vi "loopback.vi"() -> ()   [LabVIEW 2019]
uses:
  <vilib>/nican/nican.llb/ncNetAttr.ctl
panel:
  out "Output Array":string[][](table)
  in  "interface":string(combo)="CAN1"
  in  "stop":bool
  in  "Data":u8[](array[numeric])=[1, 2, 3, 4, 5, 6, 7, 8] format="%.0x"
  in  "Set RTR flag?":bool
  in  "Data Length":u32=8 max=8 format="%.0x"
  in  "Arbitration Id":u32=8 format="%.0x"
  in  "Write frame":bool
  in  "Baudrate":u32=125000
  # "Writing on CAN bus"
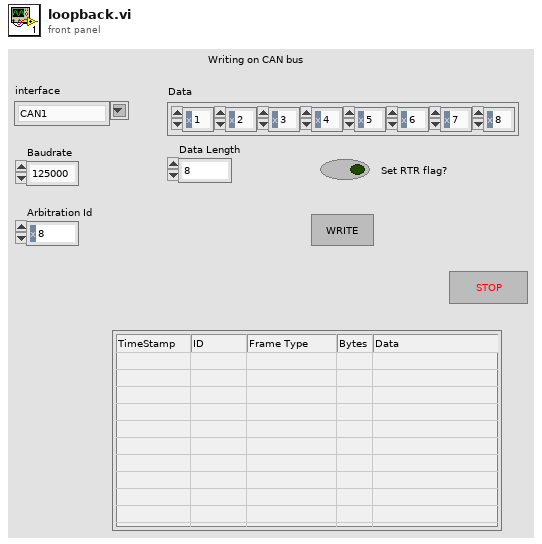
[diagram p1: front panel]
types:
  T1 = typedef "ncNetAttr.ctl" = cluster{"Start On Open":enum32{"FALSE", "TRUE"}, "Baud Rate":u32, "Read Queue Length":u32, "Write Queue Length":u32, "Standard Comparator":u32, "Standard Mask":u32, "Extended Comparator":u32, "Extended Mask":u32}
  T2 = typedef "xobjhandle.ctl" = u32
  T3 = typedef "CanFrameTimed.ctl" = cluster{"Timestamp":dbl, "ArbitrationId":u32, "IsRemote":u8, "DataLength":u8, "Data":u8[]}
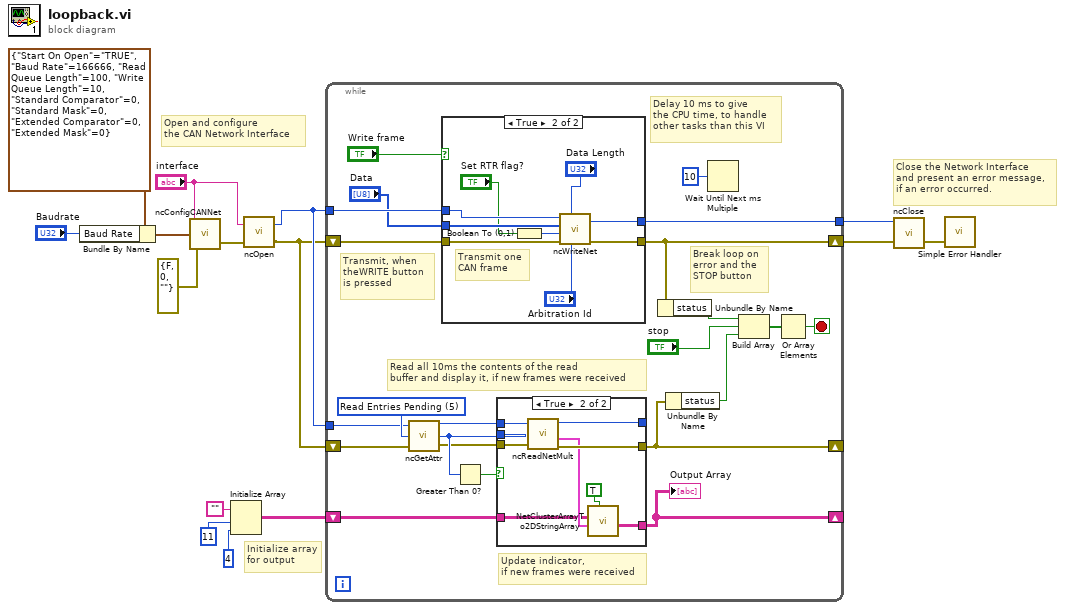
[diagram p0: block diagram]
diagram:
  # "Initialize array \nfor output"
  # "Open and configure \nthe CAN Network Interface"
  # "Close the Network Interface \nand present an error message, \nif an error occurred."
  n1 = Bundle By Name(cluster=T1 {"Start On Open"=enum."TRUE", "Baud Rate"=166666, "Read Queue Length"=100, "Write Queue Length"=10, "Standard Comparator"=0, "Standard Mask"=0, "Extended Comparator"=0, "Extended Mask"=0} ("CAN Network Interface Config"), "Baud Rate"="Baudrate") -> (w13:T1)
  n2 = call <vilib>:"ncConfigCANNet.vi"("Error in"=errorcluster {"status"=FALSE, "code"=0, "source"=""}, "CAN Network Interface Config"=w13, "ObjName"="interface") -> ("Error out"=w15:errorcluster)  [unwired: 2 in]
  n3 = Initialize Array("", 11 ("Dimension Size"), 4 ("Dimension Size")) -> (w3:string[][])
  n4 = call <vilib>:"ncOpen.vi"("Error in"=w15, "ObjName"="interface") -> ("Error out"=w1:errorcluster, "ObjHandle out"=w2:T2)
  n5 = while {
    shift-left: w1 -> [w34]
    shift-right: [w33] -> w4
    tunnel: w2 -> [w35]
    tunnel: [w36] -> w5
    shift-right: [w29] -> _
    shift-left: w3 -> [w30]
    tunnel: w2 -> [w26]
    shift-right: [w17] -> _
    shift-left: w1 -> [w25]
    stop <- w21 stop-if-true
    w28 = u32 5 items=["(reserved)", "Protocol Version", "Software Version", "Object State", "(reserved)", "Read Entries Pending", "Write Entries Pending", "ReadMult Size for Notification", "Listen Only?", "Self Reception?", "Transmit Error Counter", "Receive Error Counter", "Single Shot Transmit?", "Series 2 Filter Mode", "Series 2 Mask", "Series 2 Comparator", "Serial Number", "Form Factor", "Series", "Transceiver Type", "Interface Number", "Series 2 Error/Arb Capture", "Transceiver Mode", "Transceiver External Outputs", "Transceiver External Inputs", "Start Trigger Behavior", "Log Comm Warnings", "User RTSI Frame", "Transmit Mode", "Log Start Trigger?", "Timestamp Format", "Master Timebase Rate", "Virtual Bus Timing"] ("AttrId")
    # "Update indicator, \nif new frames were received"
    # "Read all 10ms the contents of the read \nbuffer and display it, if new frames were received"
    # "Transmit, when \ntheWRITE button \nis pressed"
    # "Delay 10 ms to give \nthe CPU time, to handle \nother tasks than this VI"
    # "Break loop on \nerror and the\nSTOP button"
    n6 = call <vilib>:"ncGetAttr.vi"("Error in"=w25, "AttrId"=w28, "ObjHandle in"=w26) -> ("Error out"=w24:errorcluster, "AttrValue"=w27:u32, "ObjHandle out"=w23:T2)
    n7 = case shown="True" "Write frame" {
      tunnel: w35 -> [w50 w59]
      tunnel: w34 -> [w51 w60]
      tunnel: [w51 w58] -> w33
      tunnel: "Data" -> [_ w57]
      tunnel: [w50 w56] -> w36
      frame False {
      }
      frame True {
        # "Transmit one \nCAN frame"
        n8 = Boolean To (0,1)(Boolean="Set RTR flag?") -> (0, 1=w55:i16)
        n9 = call <vilib>:"ncWriteNet.vi"("ArbitrationId"="Arbitration Id", "DataLength"="Data Length", "Error in"=w60, "IsRemote"=w55, "Data"=w57, "ObjHandle in"=w59) -> ("Error out"=w58:errorcluster, "ObjHandle out"=w56:T2)
      }
    }
    n10 = Greater Than 0?(x=w27) -> (x > 0?=w22:bool)
    n11 = case shown="True" w22 {
      tunnel: [w38 w49] -> w17
      tunnel: [w39 w47] -> _
      tunnel: w30 -> [w40 w46]
      tunnel: w27 -> [_ w45]
      tunnel: [w40 w43] -> w29
      tunnel: w24 -> [w38 w42]
      tunnel: w23 -> [w39 w41]
      frame False {
      }
      frame True {
        n12 = call <vilib>:"ncReadNetMult.vi"("ObjHandle in"=w41, "Requested Number of Frames"=w45, "Error in"=w42) -> ("ObjHandle out"=w47:T2, "Data"=w48:T3[], "Error out"=w49:errorcluster)  [unwired: 1 out]
        n13 = call <vilib>:"NetClusterArrayTo2DStringArray.vi"("Hexadecimal?"=TRUE, "Data from ncReadNetMult"=w48, "Input Array"=w46) -> ("Output Array"=w43:string[][])  [unwired: 8 in]
      }
    }
    "Output Array" <- w29
    n14 = Unbundle By Name(w33) -> ("status"=w20:bool)
    n15 = Unbundle By Name(w17) -> ("status"=w18:bool)
    n16 = Wait Until Next ms Multiple(millisecond multiple=u32 10) -> ()  [unwired: 1 out]
    n17 = Build Array(w20, "stop", w18) -> (w16:bool[])
    n18 = Or Array Elements(Boolean array=w16) -> (logical OR=w21:bool)
  }
  n19 = call <vilib>:"ncClose.vi"("Error in"=w4, "ObjHandle in"=w5) -> ("Error out"=w6:errorcluster)  [unwired: 1 in]
  n20 = call <vilib>:"Simple Error Handler.vi"("error in (no error)"=w6) -> ()  [unwired: 4 in, 5 out]
